vi "Query with 2D 64bit Integer Result.vi"(8 "error in (no error)":errorcluster, 10 "Query string":string, 11 "mysql in":refnum<class "mysql.lvclass">) -> (0 "error out":errorcluster, 2 "Result":i64[][](array[numeric]), 3 "mysql out":refnum<class "mysql.lvclass">)   [LabVIEW 2020, in "mysql.lvlib" / "mysql.lvclass"]
uses:
  mysql.lvclass
  54e9be2e-ce8f-4324-b773-dc371fc75995.vi
  54e9be2e-ce8f-4324-b773-dc371fc75995.vi/54f5d512-eb57-4047-a6bb-a9bcbcc7dc9e.vi
  54e9be2e-ce8f-4324-b773-dc371fc75995.vi/2e7fb4c0-86d8-4117-9d40-4bf757cfd607.vi
  private/Mysql command.vi
  private/Mysql data reader 2D I64.vi
  private/ping connection and reopen if needed.vi
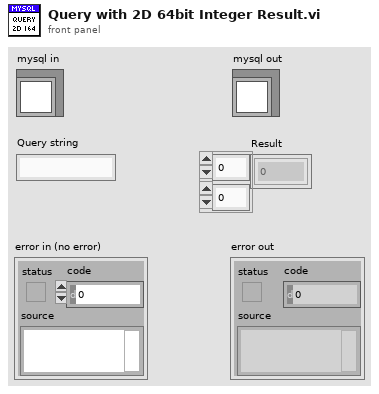
[diagram p1: front panel]
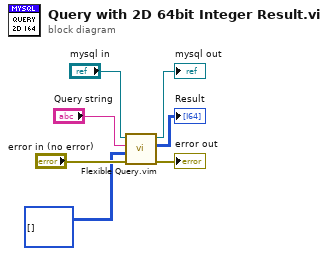
[diagram p0: block diagram]
diagram:
  n1 = call "Flexible Query.vim"("error in (no error)"="error in (no error)", "Type in"=i64[][] [] ("Result 2"), "Query string"="Query string", "mysql in"="mysql in") -> ("error out"=→"error out":errorcluster, "Result"=→"Result":i64[][], "mysql out"=→"mysql out":refnum<class "mysql.lvclass">)  [unwired: 5 in]
